vi "log_event_to_string.vi"(8 "Add newline":bool=TRUE, 11 "Log event":T1 {"Timestamp" format="%<%.3X>T"}) -> (3 "String":string)   [LabVIEW 2012]
uses:
  log_event.ctl
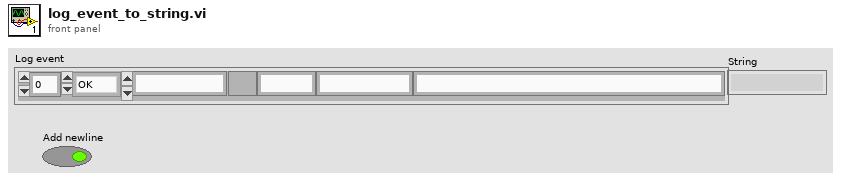
[diagram p1: front panel]
types:
  T1 = typedef "log_event.ctl" = cluster{"Facility ID":i32, "Severity":enum16{"OK", "Debug", "Warn", "Error"}, "Timestamp":timestamp, "Facility":string, "State":string, "Message":string}
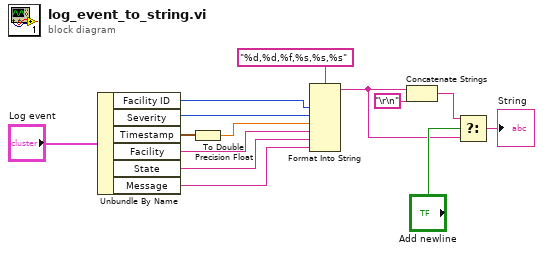
[diagram p0: block diagram]
diagram:
  n1 = Unbundle By Name("Log event") -> ("Facility ID"=w13:i32, "Severity"=w12:enum16{"OK", "Debug", "Warn", "Error"}, "Timestamp"=w7:timestamp, "Facility"=w11:string, "State"=w10:string, "Message"=w9:string)
  n2 = To Double Precision Float(number=w7) -> (double precision float=w6:dbl)
  n3 = Format Into String(format string="%d,%d,%f,%s,%s,%s", w13, w12, w6, w11, w10, w9) -> (resulting string=w3:string)  [unwired: 2 in, 1 out]
  n4 = Concatenate Strings(w3, "\r\n") -> (w2:string)
  n5 = Select(t=w2, s="Add newline", f=w3) -> (s? t:f=→"String":string)
